vi "setup_window_display.vi"(8 "error in (no error)":errorcluster) -> (0 "error out":errorcluster, 2 "Height":i16, 3 "Width":i16)   [LabVIEW 2019]
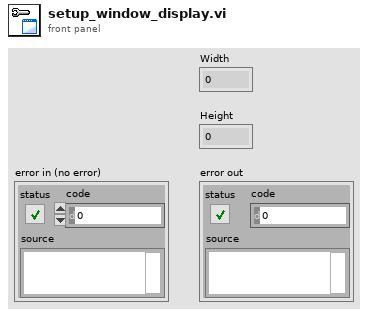
[diagram p1: front panel]
types:
  T1 = typedef "LVAllMonitorsDisplayTypeDef.ctl" = cluster{"Bounds":cluster{"Left":i16, "Top":i16, "Right":i16, "Bottom":i16}, "Depth":i16}[]
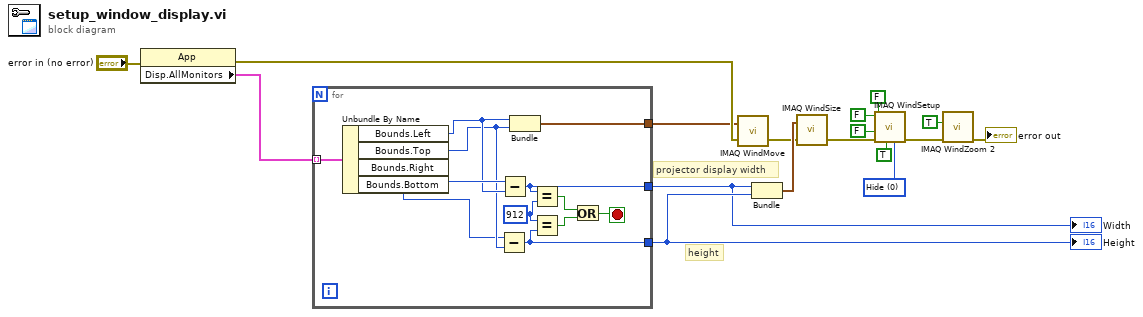
[diagram p0: block diagram]
diagram:
  w8 = 0 items=["Hide", "Show", "No change"] ("Scrollbars (No change)")
  # "height"
  # "projector display width"
  n1 = property class="App"(error in="error in (no error)") -> (error out=w16:errorcluster, "Disp.AllMonitors"=w1:T1)  [unwired: 1 in, 1 out]
  n2 = for {
    tunnel: [w22] -> w15
    tunnel: [w23] -> w14
    tunnel: [w25] -> w7
    tunnel: w1 -> [w24] mode=indexing
    stop <- w18 stop-if-true
    w21 = 912
    n3 = Unbundle By Name(w24) -> ("Bounds.Left"=w28:i16, "Bounds.Top"=w27:i16, "Bounds.Right"=w29:i16, "Bounds.Bottom"=w26:i16)
    n4 = Subtract(x=w26, y=w27) -> (x-y=w22:i16)
    n5 = Subtract(x=w29, y=w28) -> (x-y=w23:i16)
    n6 = Bundle("Left"=w28, "Top"=w27) -> (w25:cluster{"Left":i16, "Top":i16})  [unwired: 1 in]
    n7 = Equal?(x=w23, y=w21) -> (x = y?=w20:bool)
    n8 = Equal?(x=w21, y=w22) -> (x = y?=w19:bool)
    n9 = Or(x=w20, y=w19) -> (x .or. y?=w18:bool)
  }
  "Height" <- w15
  "Width" <- w14
  n10 = call "IMAQ WindMove"("Coordinates (screen)"=w7, "error in (no error)"=w16) -> ("error out"=w3:errorcluster)  [unwired: 3 in, 1 out]
  n11 = Bundle(w14, w15) -> (w5:cluster{i16, i16})  [unwired: 1 in]
  n12 = call "IMAQ WindSize"("error in (no error)"=w3, "Width & Height"=w5) -> ("error out"=w2:errorcluster)  [unwired: 4 in, 2 out]
  n13 = call "IMAQ WindSetup"("Scrollbars (No change)"=w8, "Window is floating? (No)"=TRUE, "error in (no error)"=w2, "Window has title bar? (Yes)"=FALSE, "Window can close? (Yes)"=FALSE, "Window can grow? (Yes)"=FALSE) -> ("error out"=w4:errorcluster)  [unwired: 5 in]
  n14 = call "IMAQ WindZoom 2"("error in (no error)"=w4, "Zoom to Fit? (False)"=TRUE ("Zoom to Fit? (T)")) -> ("error out"=→"error out":errorcluster)  [unwired: 6 in, 3 out]
